vi "LED_with_wait.vi"(4 "Testpulser On/Off":bool, 7 "FPGA I/O In":refnum<k21>="IO Module\\D0 0", 8 "Testpulse Time Delay (20 ns ticks)":u32=15, 9 "Testpulse Separation (20 ns ticks)":u32=500, 10 "Total number of pulses input":u64, 11 "Testpulse duration (20 ns ticks)":u32=1) -> (0 "Is Test Pulse?":bool, 2 "Total number of pulses sent":u64)   [LabVIEW 2012]
uses:
  <vilib>/eio/EIONode/EIONode.xnode
  <vilib>/rvi/eio/common/nirviEmuTemplateMethod_errors.vi
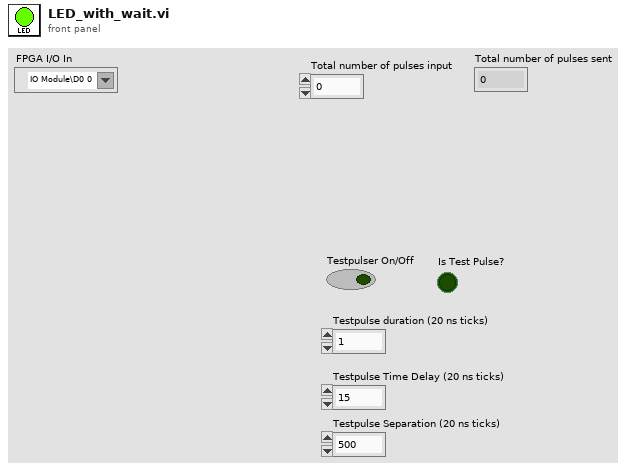
[diagram p1: front panel]
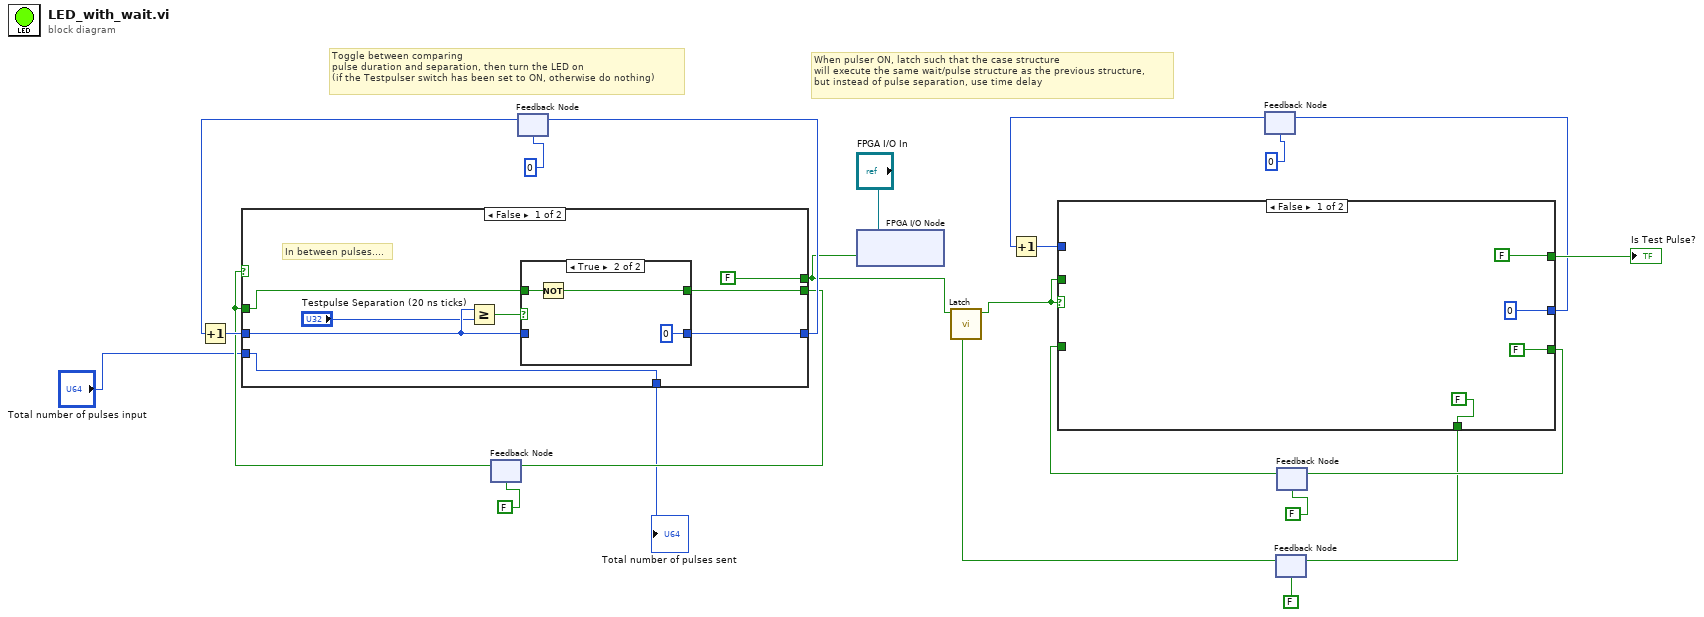
[diagram p0: block diagram]
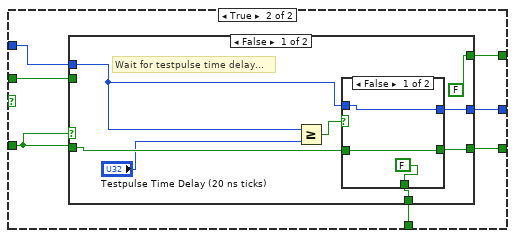
[diagram p2: hidden frame]
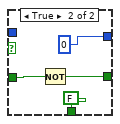
[diagram p3: hidden frame]
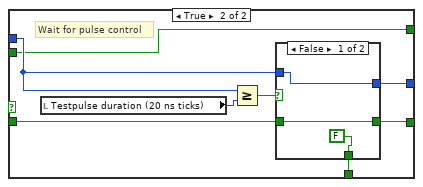
[diagram p4: hidden frame]
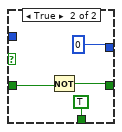
[diagram p5: hidden frame]
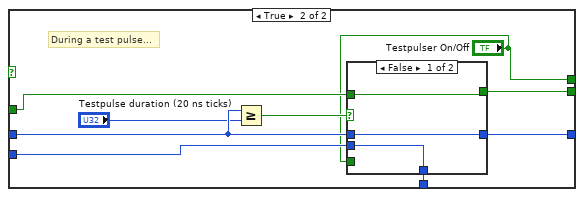
[diagram p7: hidden frame]
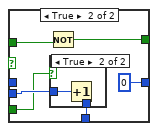
[diagram p8: hidden frame]
diagram:
  # "Toggle between comparing \npulse duration and separation, then turn the LED on\n(if the Testpulser switch has been set to ON, otherwise do nothing)"
  # "When pulser ON, latch such that the case structure\nwill execute the same wait/pulse structure as the previous structure, \nbut instead of pulse separation, use time delay"
  n1 = feedback #1(FALSE) -> (w17:bool)
  n2 = feedback #2(u32 0) -> (w20:u32)
  n3 = Increment(x=w20) -> (x+1=w23:u32)
  n4 = case shown="False" w17 {
    tunnel: w23 -> [w28 w43]
    tunnel: [w31 w44] -> w19
    tunnel: [w30 w45] -> w9
    tunnel: [FALSE ("IO Module\\D0 0") "Testpulser On/Off"] -> w4
    tunnel: w17 -> [w25 w40]
    tunnel: "Total number of pulses input" -> [w24 w39]
    tunnel: [w24 w38] -> w2
    frame False {
      # "In between pulses...."
      n5 = Greater Or Equal?(x=w28, y="Testpulse Separation (20 ns ticks)") -> (x >= y?=w27:bool)
      n6 = case shown="True" w27 {
        tunnel: [w33 u32 0] -> w31
        tunnel: w28 -> [w33 _]
        tunnel: [w32 w35] -> w30
        tunnel: w25 -> [w32 w34]
        frame False {
        }
        frame True {
          n7 = Not(x=w34) -> (.not. x?=w35:bool)
        }
      }
    }
    frame True {
      # "During a test pulse..."
      n8 = Greater Or Equal?(x=w43, y="Testpulse duration (20 ns ticks)") -> (x >= y?=w42:bool)
      n9 = case shown="False" w42 {
        tunnel: w43 -> [w48 _]
        tunnel: [w47 w54] -> w45
        tunnel: [w48 u32 0] -> w44
        tunnel: w40 -> [w47 w52]
        tunnel: w39 -> [w46 w51]
        tunnel: [w46 w50] -> w38
        tunnel: "Testpulser On/Off" -> [_ w49]
        frame False {
        }
        frame True {
          n10 = Not(x=w52) -> (.not. x?=w54:bool)
          n11 = case shown="True" w49 {
            tunnel: w51 -> [w55 w57]
            tunnel: [w55 w56] -> w50
            frame False {
            }
            frame True {
              n12 = Increment(x=w57) -> (x+1=w56:u64)
            }
          }
        }
      }
    }
  }
  "Total number of pulses sent" <- w2
  n13 = feedback-in #1(w9) -> ()
  n14 = feedback-in #2(w19) -> ()
  n15 = xnode "FPGA I/O Node"("I/O Item"=w4, "FPGA I/O In"="FPGA I/O In") -> ()  [unwired: 1 out]
  n16 = feedback #3(u32 0) -> (w15:u32)
  n17 = Increment(x=w15) -> (x+1=w14:u32)
  n18 = feedback #4(FALSE) -> (w6:bool)
  n19 = call "Latch.vi"("Reset"=w6, "Input"=w4) -> ("Output"=w5:bool)  [unwired: 9 in]
  n20 = feedback #5(FALSE) -> (w11:bool)
  n21 = case shown="False" w5 {
    tunnel: w5 -> [_ w63]
    tunnel: [FALSE w65] -> w22
    tunnel: w14 -> [_ w66]
    tunnel: [u32 0 w64] -> w13
    tunnel: w11 -> [_ w68]
    tunnel: [FALSE w67] -> w10
    tunnel: [FALSE w62] -> w7
    frame False {
    }
    frame True {
      n22 = case shown="False" w68 {
        tunnel: w68 -> [w75 w88]
        tunnel: [w74 w87] -> w67
        tunnel: w66 -> [w71 w89]
        tunnel: [FALSE w85] -> w65
        tunnel: [w72 w86] -> w64
        tunnel: w63 -> [_ w85]
        tunnel: [w69 w84] -> w62
        frame False {
          # "Wait for testpulse time delay..."
          n23 = Greater Or Equal?(x=w71, y="Testpulse Time Delay (20 ns ticks)") -> (x >= y?=w76:bool)
          n24 = case shown="False" w76 {
            tunnel: w75 -> [w79 w83]
            tunnel: [w79 w82] -> w74
            tunnel: [w78 u32 0] -> w72
            tunnel: w71 -> [w78 _]
            tunnel: [FALSE FALSE] -> w69
            frame False {
            }
            frame True {
              n25 = Not(x=w83) -> (.not. x?=w82:bool)
            }
          }
        }
        frame True {
          # "Wait for pulse control"
          n26 = local read "Testpulse duration (20 ns ticks)"() -> (w91:u32)
          n27 = Greater Or Equal?(x=w89, y=w91) -> (x >= y?=w90:bool)
          n28 = case shown="False" w90 {
            tunnel: w89 -> [w93 _]
            tunnel: w88 -> [w94 w97]
            tunnel: [w94 w96] -> w87
            tunnel: [w93 u32 0] -> w86
            tunnel: [FALSE TRUE] -> w84
            frame False {
            }
            frame True {
              n29 = Not(x=w97) -> (.not. x?=w96:bool)
            }
          }
        }
      }
    }
  }
  "Is Test Pulse?" <- w22
  n30 = feedback-in #3(w13) -> ()
  n31 = feedback-in #4(w7) -> ()
  n32 = feedback-in #5(w10) -> ()
